vi "myRIO_BRig_RT_dataExp_Tcycle_Cue1Penalty_LED.vi"() -> (2 "output_Tcycle_Cue1Penalty_LED":i32)   [LabVIEW 2014]
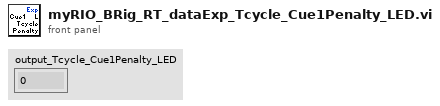
[diagram p1: front panel]
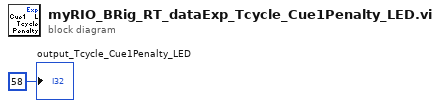
[diagram p0: block diagram]
diagram:
  "output_Tcycle_Cue1Penalty_LED" <- 58 ("output_iBlock")
